vi "FindCmdInREPL.vi"(9 "File listing":string, 11 "Command":string) -> (3 "reply":string)   [LabVIEW 2020]
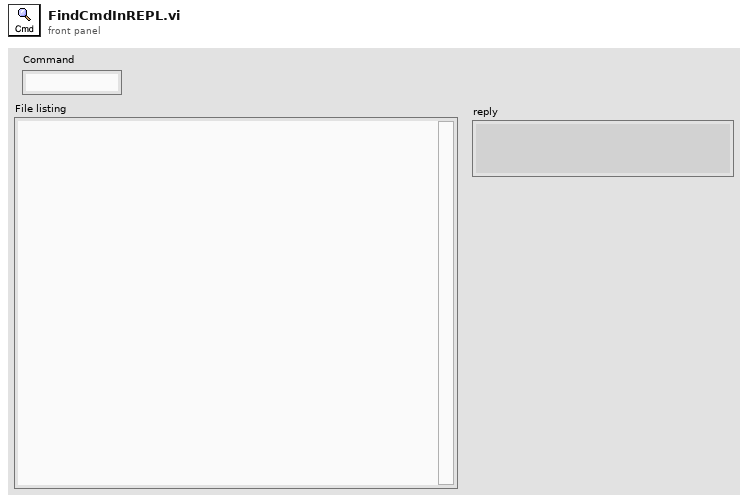
[diagram p1: front panel]
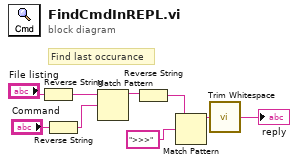
[diagram p0: block diagram]
diagram:
  # "Find last occurance"
  n1 = Reverse String(1:"File listing") -> (0:w4:string)
  n2 = Reverse String(1:"Command") -> (0:w5:string)
  n3 = Match Pattern(string=w4, regular expression=w5) -> (before substring=w2:string)  [unwired: 1 in, 3 out]
  n4 = Reverse String(1:w2) -> (0:w3:string)
  n5 = Match Pattern(string=w3, regular expression=">>>") -> (before substring=w7:string)  [unwired: 1 in, 3 out]
  n6 = call <vilib>:"Trim Whitespace.vi"("string"=w7) -> ("trimmed string"=→"reply":string)  [unwired: 1 in]
